vi "Set Mode.vi"(8 "error in (no error)":errorcluster, 10 "Mode":T1, 11 "hdl":i32) -> (0 "error out":errorcluster, 3 "hdl out":i32)   [LabVIEW 2018, in "Thorlabs_SC10.lvlib"]
uses:
  Thorlabs_SC10.lvlib
  Mode.ctl
  SC10CommandLib_x64.dll
  SC10CommandLib_win32.dll
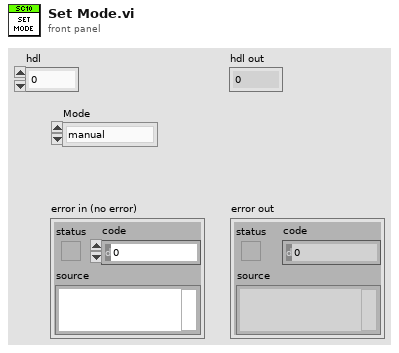
[diagram p1: front panel]
types:
  T1 = typedef "Thorlabs_SC10.lvlib/Mode.ctl" = enum16{"manual", "auto", "single", "repeat", "external gate"}
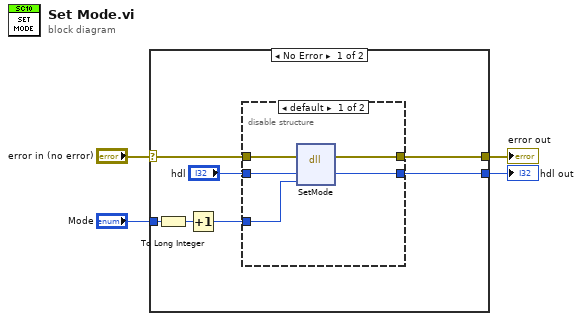
[diagram p0: block diagram]
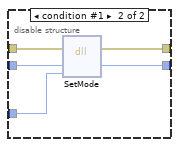
[diagram p2: hidden frame]
diagram:
  n1 = case shown="No Error" "error in (no error)" {
    selector: "error in (no error)" -> [w11 w22]
    tunnel: [w10 w22] -> w4
    tunnel: "Mode" -> [w7 _]
    tunnel: [w9 _] -> w1
    frame No Error {
      n2 = To Long Integer(number=w7) -> (32bit integer=w6:i32)
      n3 = Increment(x=w6) -> (x+1=w5:i32)
      n4 = disable-structure shown="default" {
        disable-tunnel: w11 -> [w16 w21]
        disable-tunnel: [w15 w20] -> w10
        disable-tunnel: [w14 w19] -> w9
        disable-tunnel: "hdl" -> [w13 w18]
        disable-tunnel: w5 -> [w12 w17]
        frame condition #0 (active) {
          n5 = dll-call lib="C:/Program Files (x86)/National Instruments/LabVIEW 2018/instr.lib/Thorlabs_SC10/Data/SC10CommandLib_win32.dll" fn="SetMode"(error in=w16, "hdl"=w13, "mode"=w12) -> (error out=w15:errorcluster, "hdl"=w14:i32)  [unwired: 4 in, 1 out]
        }
        frame condition #1 {
          n6 = dll-call lib="C:/Program Files/National Instruments/LabVIEW 2011/instr.lib/Thorlabs_SC10/Data/SC10CommandLib_x64.dll" fn="SetMode"(error in=w21, "hdl"=w18, "mode"=w17) -> (error out=w20:errorcluster, "hdl"=w19:i32)  [unwired: 4 in, 1 out]
        }
      }
    }
    frame Error {
    }
  }
  "error out" <- w4
  "hdl out" <- w1
